vi "Read Array of Hardware.vi"(8 "error in (no error)":errorcluster, 11 "Measurement in":refnum<class "Measurement.lvclass">) -> (0 "error out":errorcluster, 2 "Array of Hardware":refnum<class "Hardware.lvclass">[](array[class]), 3 "Measurement out":refnum<class "Measurement.lvclass">)   [LabVIEW 2015, in "Measurement Actor.lvlib" / "Measurement.lvclass"]
uses:
  Measurement.lvclass
  Hardware/Hardware.lvclass
  Measurement.lvclass/Measurement.ctl
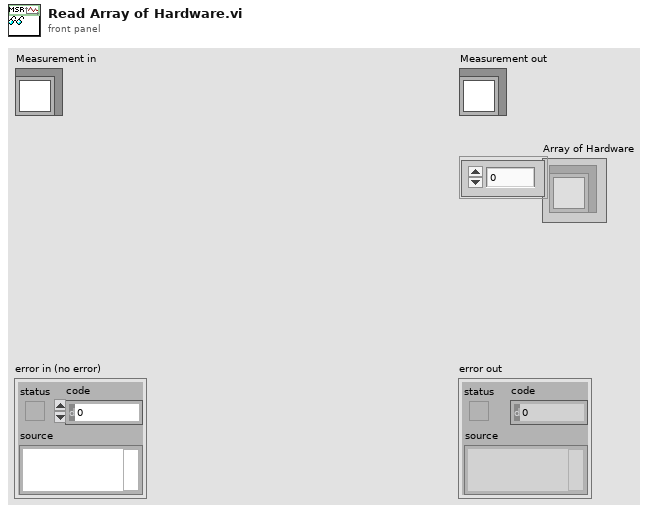
[diagram p1: front panel]
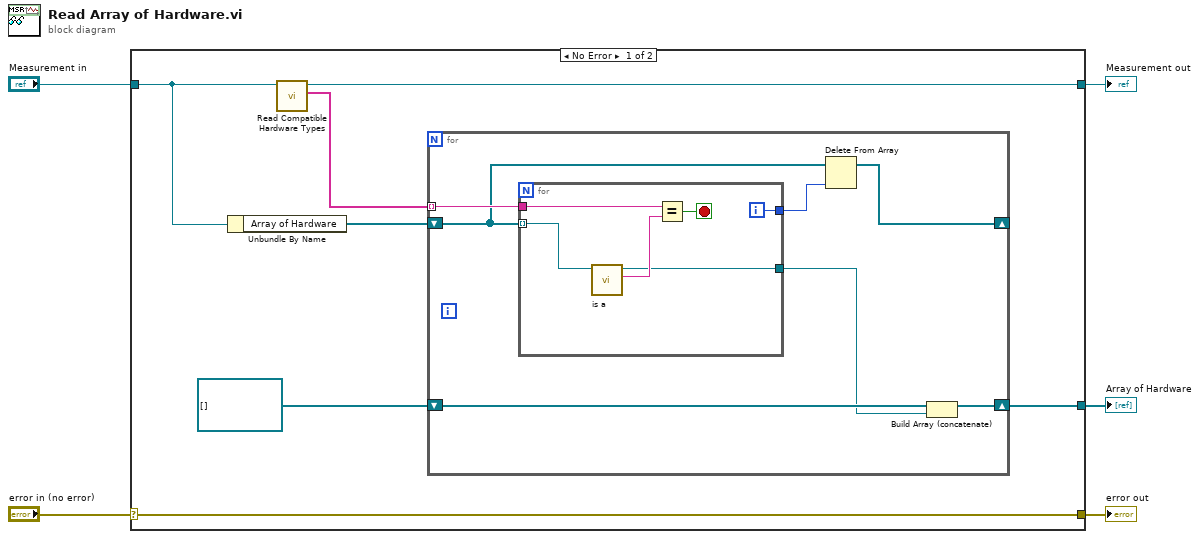
[diagram p0: block diagram]
diagram:
  n1 = case shown="No Error" "error in (no error)" {
    selector: "error in (no error)" -> [w12 w26]
    tunnel: [w12 w26] -> w4
    tunnel: [w6 w27] -> w2
    tunnel: "Measurement in" -> [w7 w27]
    tunnel: [w9 _] -> w1
    frame No Error {
      n2 = Unbundle By Name(w7) -> ("Array of Hardware"=w10:refnum<class "Hardware.lvclass">[])
      n3 = call-dynamic "Read Compatible Hardware Types.vi"("Measurement in"=w7) -> ("Compatible Hardware Types"=w8:string[], "Measurement out"=w6:refnum<class "Measurement.lvclass">)  [unwired: 8 in, 1 out]
      n4 = for {
        tunnel: w8 -> [w19] mode=indexing
        shift-right: [w17] -> w9
        shift-left: refnum<class "Hardware.lvclass">[] [] ("Array of Hardware") -> [w18]
        shift-right: [w13] -> _
        shift-left: w10 -> [w15]
        n5 = for {
          tunnel: w19 -> [w24]
          tunnel: w15 -> [w25] mode=indexing
          tunnel: [w22] -> w16
          tunnel: [w20] -> w14
          i -> [w20]
          stop <- w21 stop-if-true
          n6 = call-dynamic "is a.vi"("Hardware in"=w25) -> ("is a"=w23:string, "Hardware out"=w22:refnum<class "Hardware.lvclass">)  [unwired: 8 in, 1 out]
          n7 = Equal?(x=w24, y=w23) -> (x = y?=w21:bool)
        }
        n8 = Delete From Array(array=w15, index=w14) -> (array with subset deleted=w13:refnum<class "Hardware.lvclass">[])  [unwired: 1 in, 1 out]
        n9 = Build Array (concatenate)(w18, w16) -> (w17:refnum<class "Hardware.lvclass">[])
      }
    }
    frame Error {
    }
  }
  "error out" <- w4
  "Measurement out" <- w2
  "Array of Hardware" <- w1
